vi "Update Tag Details.vi"(8 "Error In":errorcluster, 10 "Commit Info":string, 11 "Git-Api In":refnum<class "GIT-api.lvclass">) -> (0 "Error Out":errorcluster, 3 "Updated Commit Info":string)   [LabVIEW 2016]
doc: "Update the latest tag details (if exists) in the <B>Commit Info</B>."
uses:
  <vilib>/Hampel Software Engineering/Git API/Git API/GIT-api.lvclass
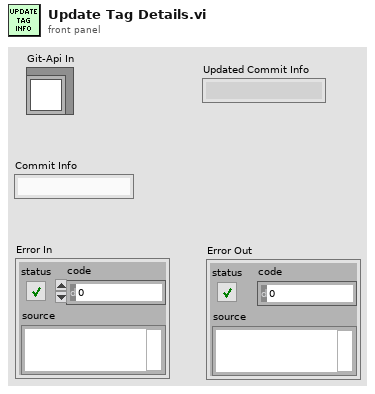
[diagram p1: front panel]
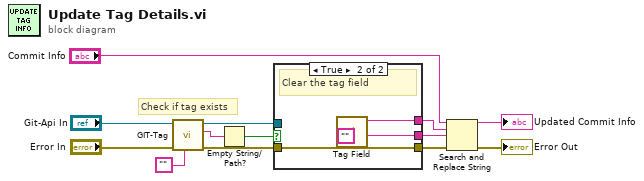
[diagram p0: block diagram]
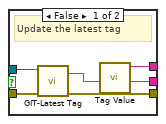
[diagram p2: hidden frame]
diagram:
  # "Check if tag exists"
  n1 = call <vilib>:"GIT-Tag.vi"("param"="", "error in"="Error In", "git-api in"="Git-Api In") -> ("error out"=w6:errorcluster, "std out"=w1:string, "git-api out"=w4:refnum<class "GIT-api.lvclass">)  [unwired: 6 in]
  n2 = Empty String/Path?(string/path=w1) -> (empty?=w3:bool)
  n3 = case shown="True" w3 {
    tunnel: [w14 w19] -> w10
    tunnel: [w18 ""] -> w9
    tunnel: w6 -> [w17 w20]
    tunnel: [w16 w20] -> w5
    tunnel: w4 -> [w15 _]
    frame False {
      # "Update the latest tag"
      n4 = call <vilib>:"GIT-Latest Tag.vi"("error in"=w17, "git-api in"=w15) -> ("error out"=w16:errorcluster, "Latest Tag"=w18:string)  [unwired: 6 in, 2 out]
      n5 = call "Tag Value.vi"() -> ("Tag Value"=w14:string)  [unwired: 11 in]
    }
    frame True {
      # "Clear the tag field"
      n6 = call "Tag Field.vi"() -> ("Tag Field"=w19:string)  [unwired: 11 in]
    }
  }
  n7 = Search and Replace String(input string="Commit Info", search string=w10, replace string=w9, error in=w5) -> (result string=→"Updated Commit Info":string, error out=→"Error Out":errorcluster)  [unwired: 4 in, 2 out]
